vi "Untitled 3.vi"   [LabVIEW 2017]
uses:
  <vilib>/gpm_packages/@cs/mva-core/Source/MonitoredMediator/MonitoredMediator/MonitoredMediator.lvclass
  C:/Program Files/National Instruments/LabVIEW 2017/vi.lib/gpm_packages/@cs/mva-core/Source/IMediator/IMediator/IMediator.lvclass
  C:/Program Files/National Instruments/LabVIEW 2017/vi.lib/ActorFramework/Actor/Actor.lvclass
  <vilib>/gpm_packages/@cs/BusMonitor/ListboxBusMonitor/ListboxBusMonitor/ListboxBusMonitor.lvclass/ListboxBusMonitor.ctl
  <vilib>/gpm_packages/@cs/mva-core/Source/IMediator/PublishRequest/PublishRequest.lvclass
  <vilib>/gpm_packages/@cs/event-logger/Source/Composed Log/LoggerReference/LoggerReference.lvclass
  <vilib>/gpm_packages/@cs/mva-core/Source/MonitoredMediator/MonitoredMediator/MonitoredMediator.lvclass/MonitoredMediator.ctl
  <vilib>/gpm_packages/@cs/mva-core/Source/IMediator/IMediator/IMediator.lvclass/IMediator.ctl
  <vilib>/gpm_packages/@cs/mva-core/Source/IMediator/PublishRequest/PublishRequest.lvclass/PublishRequest.ctl
  <vilib>/gpm_packages/@cs/mva-core/Source/IMediator/IMediator Messages/Publish Msg/Publish Msg.lvclass/Publish Msg.ctl
  <vilib>/gpm_packages/@cs/actor-framework-messages/Source/RoundTripMessage/RoundTripMessage.lvclass/RoundTripMessage.ctl
  <vilib>/ActorFramework/Message Enqueuer/Message Enqueuer.lvclass/Message Enqueuer.ctl
  855b1a76-252b-4ab3-b60a-012205ba5076.vi
  <vilib>/gpm_packages/@cs/mva-core/Source/MonitoredMediator/MonitoredMediator/Private Write BusMonitors.vi
  <vilib>/gpm_packages/@cs/actor-framework-messages/Source/RoundTripMessage/Return Round-Trip Message.vi
  <vilib>/ActorFramework/Message Enqueuer/Enqueue.vi
  <vilib>/gpm_packages/@cs/mva-core/Source/IMediator/IMediator Messages/Publish Msg/Publish Msg.lvclass
  C:/Program Files/National Instruments/LabVIEW 2017/vi.lib/gpm_packages/@cs/actor-framework-messages/Source/RoundTripMessage/RoundTripMessage.lvclass
  <vilib>/gpm_packages/@cs/actor-framework-messages/Source/RoundTripMessage/RoundTripMessage.lvclass
  C:/Program Files/National Instruments/LabVIEW 2017/vi.lib/ActorFramework/Message/Message.lvclass
  <vilib>/ActorFramework/Stop Msg/Stop Msg.lvclass
  <vilib>/Utility/error.llb/Error Cluster From Error Code.vi
  <vilib>/ActorFramework/Message Priority Queue/Priority Enqueue.vi
  <vilib>/gpm_packages/@cs/BusMonitor/ListboxBusMonitor/ListboxBusMonitor/ListboxBusMonitor.lvclass
  <vilib>/gpm_packages/@cs/mva-core/Source/IMediator/IMediator/IMediator.lvclass
  <vilib>/ActorFramework/Actor/Actor.lvclass
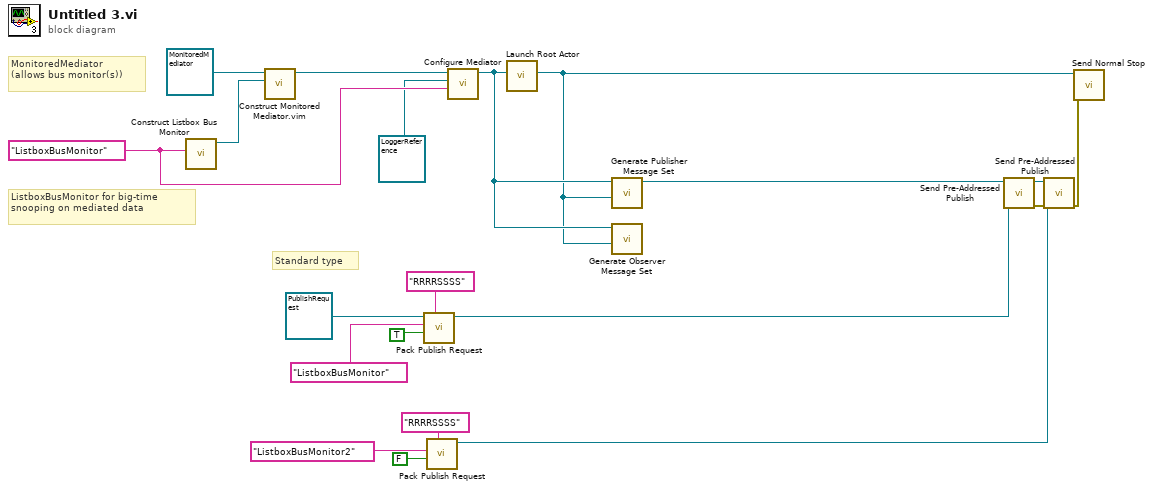
[diagram p0: block diagram]
diagram:
  w9 = "ListboxBusMonitor" ("Show Panel Boolean Name")
  # "Standard type"
  # "ListboxBusMonitor for big-time\nsnooping on mediated data"
  # "MonitoredMediator\n(allows bus monitor(s))"
  n1 = call <vilib>:"Construct Listbox Bus Monitor.vi"("Show Panel Boolean Name"=w9) -> ("ListboxBusMonitor out"=w18:refnum<class "ListboxBusMonitor.lvclass">)  [unwired: 10 in]
  n2 = call "Construct Monitored Mediator.vim"("Startup Bus Monitor(s)"=w18, "MonitoredMediator in"=refnum<class "MonitoredMediator.lvclass"> refnum ("MonitoredMediator.lvlib:MonitoredMediator.lvclass")) -> ("MonitoredMediator out"=w17:refnum<class "MonitoredMediator.lvclass">)  [unwired: 9 in]
  n3 = call <vilib>:"Pack Publish Request.vi"("Publisher ID"="RRRRSSSS", "Value"=TRUE, "Datum Name"="ListboxBusMonitor", "PublishRequest In"=refnum<class "PublishRequest.lvclass"> refnum) -> ("PublishRequest Out"=w14:refnum<class "PublishRequest.lvclass">)  [unwired: 6 in, 1 out]
  n4 = call <vilib>:"Pack Publish Request.vi"("Publisher ID"="RRRRSSSS", "Value"=FALSE, "Datum Name"="ListboxBusMonitor2") -> ("PublishRequest Out"=w6:refnum<class "PublishRequest.lvclass">)  [unwired: 7 in, 1 out]
  n5 = call <vilib>:"Configure Mediator.vi"("Framework Instance Alias"=w9, "Event Log Instance"=refnum<class "LoggerReference.lvclass"> refnum, "Mediator in"=w17) -> ("Mediator out"=w16:refnum<class "MonitoredMediator.lvclass">)  [unwired: 8 in]
  n6 = call <vilib>:"Launch Root Actor.vi"("Actor"=w16) -> ("Actor's Enqueuer"=w10:refnum<class "Message Enqueuer.lvclass">)  [unwired: 9 in, 1 out]
  n7 = call-dynamic "Generate Publisher Message Set.vi"("Mediator Enqueuer"=w10, "IMediator in"=w16) -> ("Publish Msg"=w3:refnum<class "Publish Msg.lvclass">)  [unwired: 7 in, 2 out]
  n8 = call-dynamic "Generate Observer Message Set.vi"("Mediator Enqueuer"=w10, "Mediator Type"=w16) -> ()  [unwired: 8 in, 2 out]
  n9 = call <vilib>:"Send Pre-Addressed Publish.vi"("PublishRequest"=w14, "Publish Message"=w3) -> ("error out"=w1:errorcluster)  [unwired: 9 in]
  n10 = call <vilib>:"Send Pre-Addressed Publish.vi"("error in (no error)"=w1, "PublishRequest"=w6, "Publish Message"=w3) -> ("error out"=w2:errorcluster)  [unwired: 8 in]
  n11 = call <vilib>:"Send Normal Stop.vi"("error in (no error)"=w2, "Message Enqueuer"=w10) -> ()  [unwired: 9 in, 1 out]
